vi "FindFaces.vi"() -> ()   [LabVIEW 2018]
panel:
  out "Image to process":picture
  out "Processed image":picture
  out "Error":errorcluster
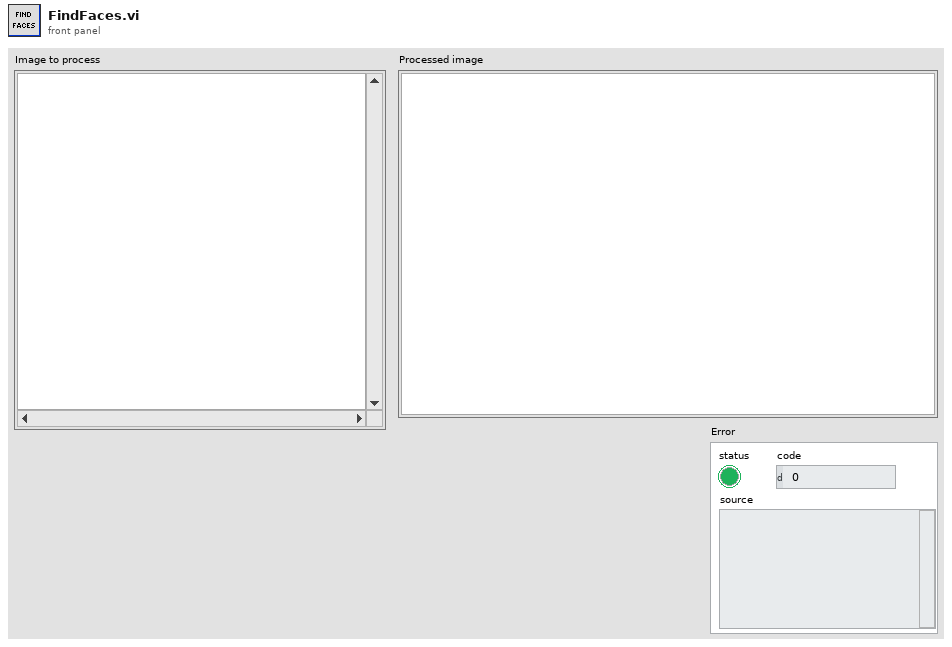
[diagram p1: front panel]
types:
  T1 = typedef "imagedata.ctl" = cluster{"image type":i32, "image depth":i32, "image":u8[], "mask":u8[], "colors":u32[], "Rectangle":cluster{"left":i16, "top":i16, "right":i16, "bottom":i16}}
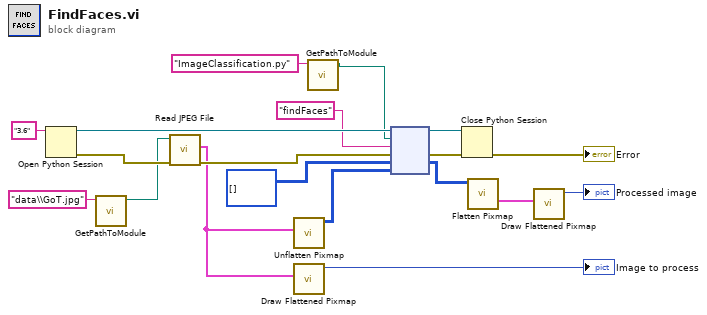
[diagram p0: block diagram]
diagram:
  n1 = Open Python Session(python version="3.6" ("Python version")) -> (session out=w19:refnum<k35>, error out=w11:errorcluster)  [unwired: 2 in]
  n2 = call "GetPathToModule.vi"("module name"="data\\GoT.jpg") -> ("path to module"=w1:path)  [unwired: 10 in]
  n3 = call <vilib>:"Read JPEG File.vi"("error in (no error)"=w11, "path to JPEG file"=w1) -> ("error out"=w10:errorcluster, "image data"=w8:T1)  [unwired: 7 in, 1 out]
  n4 = call <vilib>:"Unflatten Pixmap.vi"("image data"=w8) -> ("24-bit pixmap"=w5:u32[][])  [unwired: 4 in, 6 out]
  n5 = call <vilib>:"Draw Flattened Pixmap.vi"("image data"=w8) -> ("new picture"=→"Image to process":picture)  [unwired: 8 in]
  n6 = call "GetPathToModule.vi"("module name"="ImageClassification.py") -> ("path to module"=w3:path)  [unwired: 10 in]
  n7 = node(w19, w3, "findFaces" ("function name"), w10, u32[][] [], w5) -> (w18:refnum<k35>, w17:errorcluster, w6:u32[][])  [unwired: 1 in, 2 out]
  n8 = Close Python Session(session in=w18, error in=w17) -> (11:→"Error":errorcluster)
  n9 = call <vilib>:"Flatten Pixmap.vi"("24-bit pixmap"=w6) -> ("image data"=w13:T1)  [unwired: 10 in]
  n10 = call <vilib>:"Draw Flattened Pixmap.vi"("image data"=w13) -> ("new picture"=→"Processed image":picture)  [unwired: 8 in]
